vi "Failures.vi"(1 "TestResult In":refnum<class "TestResult.lvclass">) -> (0 "Failures":refnum<class "TestFailure.lvclass">[](array[class]))   [LabVIEW 2019, in "TestResult.lvclass"]
doc: "Returns the list of failures."
uses:
  TestResult.lvclass
  TestFailure/TestFailure.lvclass
  TestResult.lvclass/TestResult.ctl
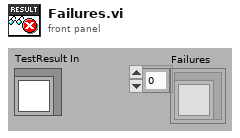
[diagram p1: front panel]
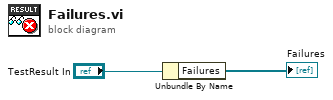
[diagram p0: block diagram]
diagram:
  n1 = Unbundle By Name("TestResult In") -> ("Failures"=→"Failures":refnum<class "TestFailure.lvclass">[])
